vi "PGPASS.Select Connection.vi"(8 "error in":errorcluster, 11 "search string":string) -> (0 "error out":errorcluster, 3 "connection string":string)   [LabVIEW 2019, in "PGPASS.lvlib"]
doc: "Searches the PGPASS file for the connection given by <b>search string</b>. You must provide at least the minimum amount of information needed to discriminate entries in the PGPASS file.\n\nIf your file contains two entries:\n\n1.234.56.789:5432:db1:user1:***\n1.234.56.789:5432:db1:user2:***\n\n\"user = user1\" would be a sufficient search string.\n\n<b>keywords</b>: host, port, dbname, user\n\n<b>note</b>: passwords must be saved in the PGPASS file. LabVIEW will not attempt to read or display them; they will be handled by pqlib."
uses:
  PGPASS.lvlib
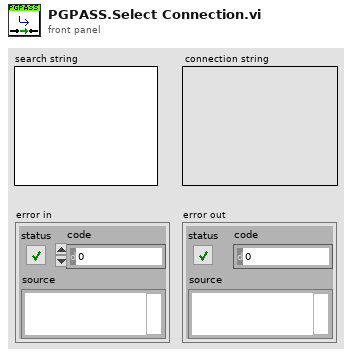
[diagram p1: front panel]
types:
  T1 = typedef "PGPASS.lvlib/PGPASS.Connection Information.ctl" = cluster{"host":string, "port":string, "dbname":string, "user":string, "password":string}
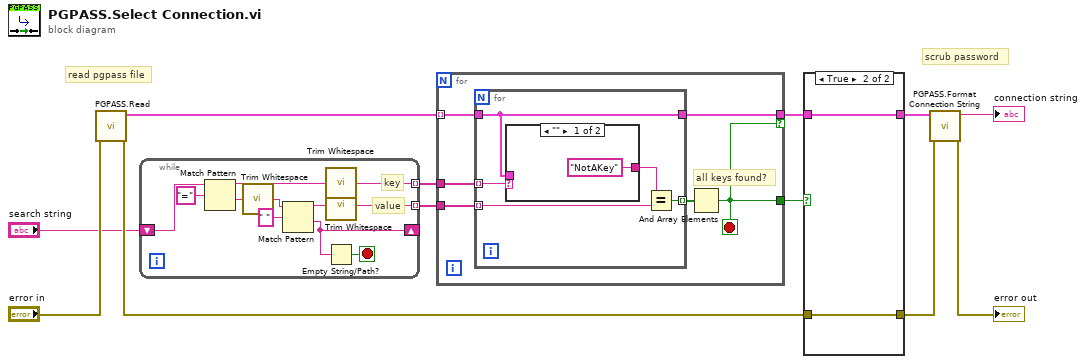
[diagram p0: block diagram]
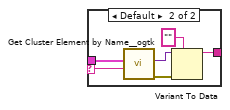
[diagram p2: hidden frame]
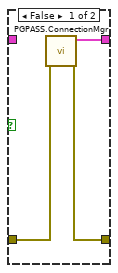
[diagram p3: hidden frame]
diagram:
  # "scrub password"
  # "read pgpass file"
  n1 = call "PGPASS.Read.vi"("error in"="error in") -> ("error out"=w8:errorcluster, "Connections"=w3:T1[])  [unwired: 9 in]
  n2 = while {
    shift-right: [w16] -> _
    shift-left: "search string" -> [w23]
    tunnel: [w20] -> w7 mode=indexing
    tunnel: [w17] -> w2 mode=indexing
    stop <- w13 stop-if-true
    # "value"
    # "key"
    n3 = Match Pattern(string=w23, regular expression="=") -> (before substring=w22:string, after substring=w15:string)  [unwired: 1 in, 2 out]
    n4 = call <vilib>:"Trim Whitespace.vi"("string"=w15) -> ("trimmed string"=w14:string)  [unwired: 1 in]
    n5 = Match Pattern(string=w14, regular expression=" ") -> (before substring=w18:string, after substring=w16:string)  [unwired: 1 in, 2 out]
    n6 = call <vilib>:"Trim Whitespace.vi"("string"=w22) -> ("trimmed string"=w20:string)  [unwired: 1 in]
    n7 = call <vilib>:"Trim Whitespace.vi"("string"=w18) -> ("trimmed string"=w17:string)  [unwired: 1 in]
    n8 = Empty String/Path?(string/path=w16) -> (empty?=w13:bool)
  }
  n9 = for {
    tunnel: [w24] -> w1
    tunnel: w3 -> [w29] mode=indexing
    tunnel: [w28] -> w6 if=w24
    tunnel: w7 -> [w27]
    tunnel: w2 -> [w26]
    stop <- w24 stop-if-true
    # "all keys found?"
    n10 = for {
      tunnel: w29 -> [w32]
      tunnel: w27 -> [w30] mode=indexing
      tunnel: w26 -> [w33] mode=indexing
      tunnel: [w32] -> w28
      tunnel: [w31] -> w25 mode=indexing
      n11 = case shown="\"\"" w30 {
        selector: w30 -> [_ w36]
        tunnel: ["NotAKey" w38] -> w34
        tunnel: w32 -> [_ w37]
        frame "" {
        }
        frame Default {
          n12 = call <userlib>:"Get Cluster Element by Name__ogtk.vi"("Element Name"=w36, "Cluster"=w37) -> ("error out"=w41:errorcluster, "VElement"=w40:variant)  [unwired: 7 in, 1 out]
          n13 = Variant To Data(error in=w41, type="", Variant=w40) -> (data=w38:string)  [unwired: 1 out]
        }
      }
      n14 = Equal?(x=w34, y=w33) -> (x = y?=w31:bool)
    }
    n15 = And Array Elements(Boolean array=w25) -> (logical AND=w24:bool)
  }
  n16 = case shown="True" w1 {
    tunnel: w8 -> [w44 w46]
    tunnel: [w43 w46] -> w11
    tunnel: w6 -> [_ w45]
    tunnel: [w42 w45] -> w5
    frame False {
      n17 = call "PGPASS.ConnectionMgr.vi"("error in (no error)"=w44) -> ("error out"=w43:errorcluster, "Connection"=w42:T1)  [unwired: 9 in]
    }
    frame True {
    }
  }
  n18 = call "PGPASS.Format Connection String.vi"("error in"=w11, "Connection Information"=w5) -> ("error out"=→"error out":errorcluster, "connection string"=→"connection string":string)  [unwired: 8 in]
